vi "_Test_Signal_Tree.vi"() -> ()   [LabVIEW 2023]
uses:
  System Explorer/Vires VTD System Explorer.lvlib
panel:
  out "RDB Signalname":string
  out "RDB Receive Objects":string caption="RDB Object Name"
  out "Tag":string
  in  "stop":bool
  in  "Tree":string(tree)
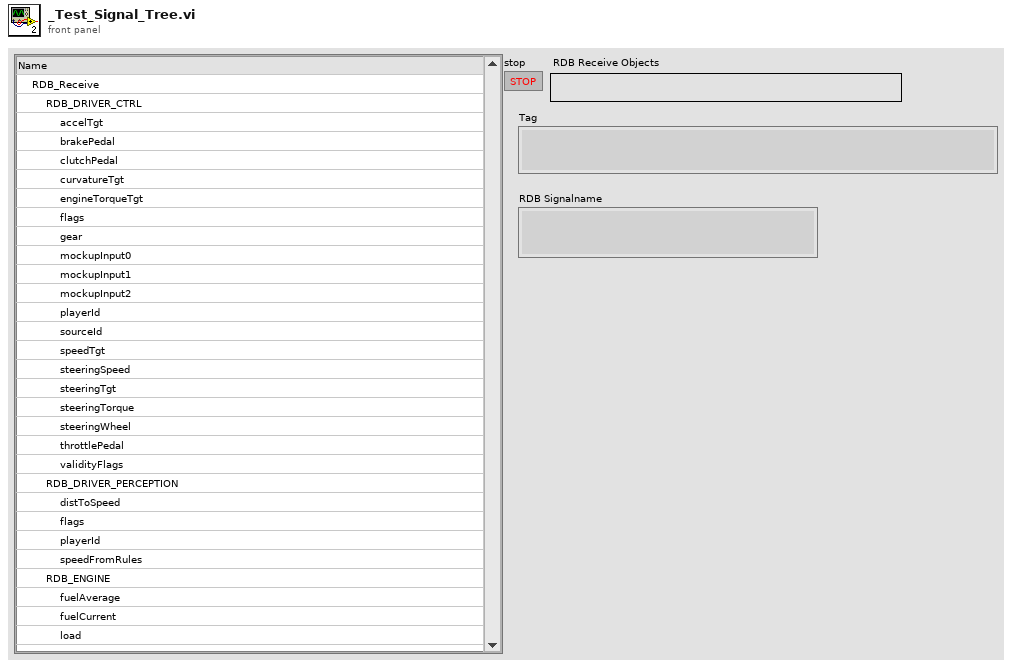
[diagram p1: front panel]
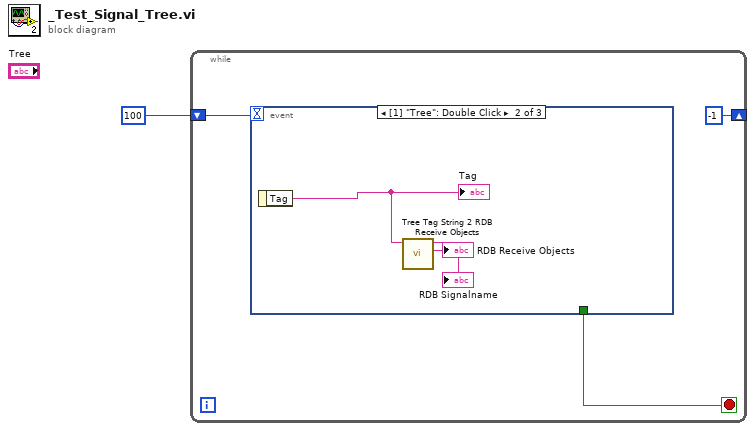
[diagram p0: block diagram]
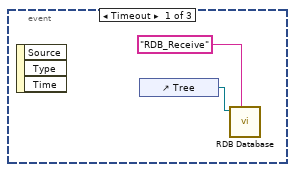
[diagram p2: hidden frame]
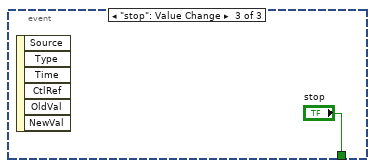
[diagram p3: hidden frame]
diagram:
  n1 = while {
    shift-right: [-1] -> _
    shift-left: 100 -> [w4]
    stop <- w2 stop-if-true
    n2 = event shown="[1] \"Tree\": Double Click" {
      selector: _ -> [_ _ _]
      dyn-events: _ -> [_ _ _]
      timeout: w4 -> [_ _ _]
      tunnel: [_ _ "stop"] -> w2
      event Timeout {
        n3 = event-data() -> ()  [unwired: 1 in, 3 out]
        n4 = control-ref of="Tree"() -> (w6:refnum<vi>)
        n5 = call "RDB Database.vi"("Filter Cluster"="RDB_Receive", "reference in"=w6) -> ()  [unwired: 8 in, 2 out]
      }
      event "Tree": Double Click {
        n6 = event-data() -> ("Tag"=w9:string)  [unwired: 1 in]
        "Tag" <- w9
        n7 = call "Tree Tag String 2 RDB Receive Objects.vi"("tag string"=w9) -> ("RDB Receive Objects"=→"RDB Receive Objects":string, "RDB Signalname"=→"RDB Signalname":string)  [unwired: 9 in]
      }
      event "stop": Value Change {
        n8 = event-data() -> ()  [unwired: 1 in, 6 out]
      }
    }
  }
